vi "Set Vehicle Position.vi"(8 "error in (no error)":errorcluster, 10 "Wash Steps":T1, 11 "Car Wash Controller in":refnum<class "Car Wash Controller.lvclass">) -> (0 "error out":errorcluster, 3 "Car Wash Controller out":refnum<class "Car Wash Controller.lvclass">)   [LabVIEW 2019, in "Car Wash Controller.lvlib" / "Car Wash Controller.lvclass"]
uses:
  Car Wash Controller.lvclass
  Vehicle Position Simulation Actor/Vehicle Position Simulation Actor Messages/Write Vehicle Position Msg/Write Vehicle Position Msg.lvclass
  Wash Steps.ctl
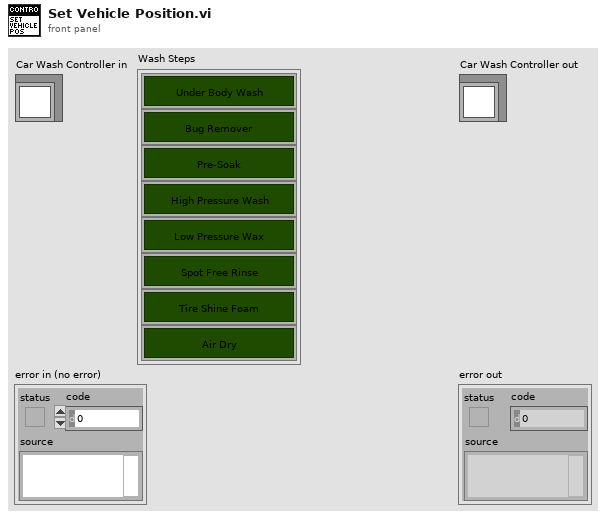
[diagram p1: front panel]
types:
  T1 = typedef "Car Wash Controller.lvlib/Car Wash Controller.lvclass/Wash Steps.ctl" = cluster{"Under Body Wash":bool, "Bug Remover":bool, "Pre-Soak":bool, "High Pressure Wash (Default)":bool, "Low Pressure Wax":bool, "Spot Free Rinse":bool, "Tire Shine Foam":bool, "Air Dry":bool}
  T2 = typedef "Car Wash Controller.lvlib/Car Wash Controller.lvclass/Staion_Wash Step_timing List.ctl" = string[][]
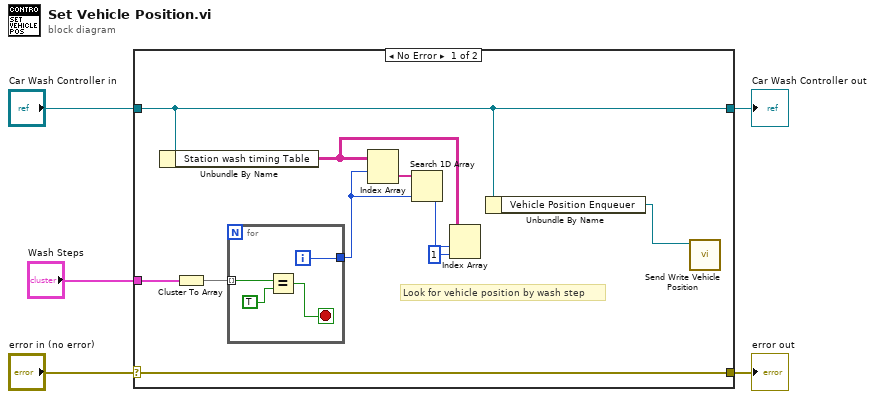
[diagram p0: block diagram]
diagram:
  n1 = case shown="No Error" "error in (no error)" {
    selector: "error in (no error)" -> [w15 w21]
    tunnel: [w15 w21] -> w4
    tunnel: [w13 w20] -> w2
    tunnel: "Car Wash Controller in" -> [w13 w20]
    tunnel: "Wash Steps" -> [w12 _]
    frame No Error {
      # "Look for vehicle position by wash step"
      n2 = Unbundle By Name(w13) -> ("Station wash timing Table"=w7:T2)
      n3 = Cluster To Array(cluster=w12) -> (array=w11:bool[])
      n4 = for {
        tunnel: w11 -> [w19] mode=indexing
        tunnel: [w16] -> w9
        i -> [w16]
        stop <- w17 stop-if-true
        n5 = Equal?(x=w19, y=TRUE) -> (x = y?=w17:bool)
      }
      n6 = Index Array(array=w7, index (row)=w9) -> (element=w10:string[])  [unwired: 1 in]
      n7 = Search 1D Array(1D array=w10, start index (0)=w9) -> (index of element=w8:i32)  [unwired: 1 in]
      n8 = Index Array(array=w7, index (row)=w8, index (col)=1 ("disabled index (col)")) -> ()  [unwired: 1 out]
      n9 = Unbundle By Name(w13) -> ("Vehicle Position Enqueuer"=w14:refnum<class "Message Enqueuer.lvclass">)
      n10 = call "Send Write Vehicle Position.vi"("Message Enqueuer"=w14) -> ()  [unwired: 9 in, 2 out]
    }
    frame Error {
    }
  }
  "error out" <- w4
  "Car Wash Controller out" <- w2
